vi "Get_Dist_from_ID.vi"(8 "error in (no error)":errorcluster, 10 "Tag":string, 11 "localDists":refnum<class "IB_DistPart.lvclass">[](array[class])) -> (0 "error out":errorcluster, 2 "index":i32, 3 "dist":refnum<class "IB_DistPart.lvclass">)   [LabVIEW 2020, in "IB_DistPart.lvclass"]
uses:
  <vilib>/AppBuilder/IB_Classes/DistPart/IB_DistPart.lvclass
  <vilib>/AppBuilder/IB_Classes/DistPart/IB_DistPart.lvclass/IB_DistPart.ctl
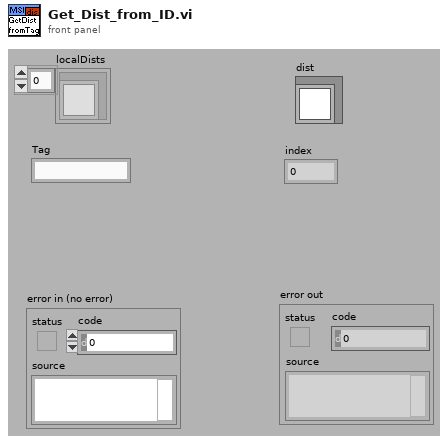
[diagram p1: front panel]
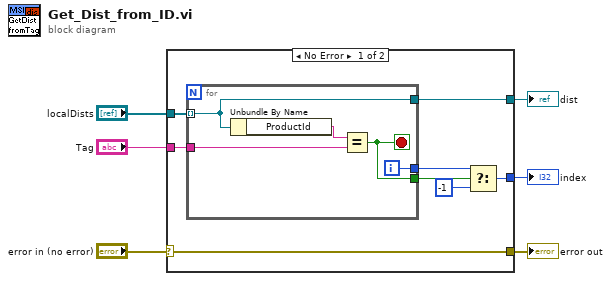
[diagram p0: block diagram]
diagram:
  n1 = case shown="No Error" "error in (no error)" {
    selector: "error in (no error)" -> [w7 w20]
    tunnel: "Tag" -> [w14 _]
    tunnel: "localDists" -> [w13 _]
    tunnel: [w12 _] -> w4
    tunnel: [w8 _] -> w3
    tunnel: [w7 w20] -> w1
    frame No Error {
      n2 = for {
        tunnel: w13 -> [w17] mode=indexing
        tunnel: w14 -> [w18]
        tunnel: [w17] -> w12
        tunnel: [w16] -> w9
        tunnel: [w15] -> w10
        i -> [w16]
        stop <- w15 stop-if-true
        n3 = Unbundle By Name(w17) -> ("ProductId"=w19:string)
        n4 = Equal?(x=w19, y=w18) -> (x = y?=w15:bool)
      }
      n5 = Select(t=w9, s=w10, f=-1) -> (s? t:f=w8:i32)
    }
    frame Error {
    }
  }
  "dist" <- w4
  "error out" <- w1
  "index" <- w3
